vi "Log Result.vi"(8 "error in (no error)":errorcluster, 10 "tdms file":refnum<k34>, 11 "Scaled I32 Array Result in":refnum<class "Scaled I32 Array Result.lvclass">) -> (0 "error out":errorcluster, 2 "tdms file out":refnum<k34>, 3 "Scaled I32 Array Result out":refnum<class "Scaled I32 Array Result.lvclass">)   [LabVIEW 2015, in "Scaled I32 Array Result.lvclass"]
uses:
  Scaled I32 Array Result.lvclass
  Scaled I32 Array Result.lvclass/Scaled I32 Array Result.ctl
  Mag Lab Result.lvclass/Mag Lab Result.ctl
  Read Scale Array.vi
  Read Group Name.vi
  Read Channel names.vi
  Read I32 Array.vi
  <vilib>/Utility/tdmsutil.llb/TDMS Create Scaling Information (Linear).vi
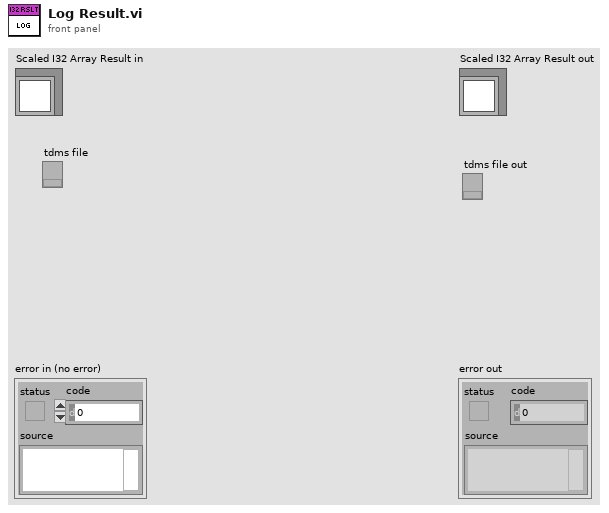
[diagram p1: front panel]
types:
  T1 = cluster{"Numeric":dbl, "Numeric":dbl, "input source":i32}
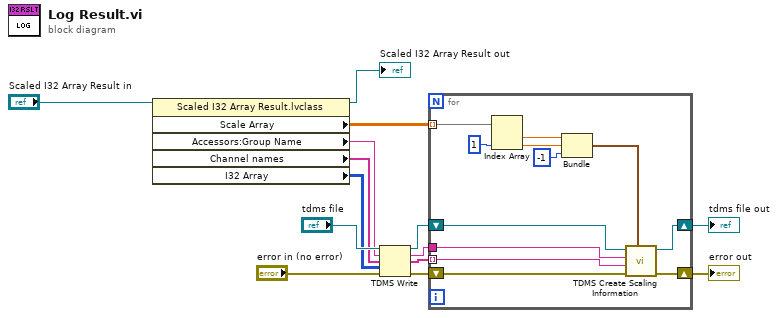
[diagram p0: block diagram]
diagram:
  n1 = property class="Scaled I32 Array Result.lvclass"(reference="Scaled I32 Array Result in") -> (reference out=→"Scaled I32 Array Result out":refnum<class "Scaled I32 Array Result.lvclass">, "Scale Array"=w5:dbl[][], "Accessors:Group Name"=w8:string, "Channel names"=w6:string[], "I32 Array"=w7:i32[][])  [unwired: 1 in, 1 out]
  n2 = TDMS Write(0:"tdms file", 5:w8, 7:w6, 9:w7, 11:"error in (no error)") -> (4:w4:refnum<k34>, 6:w9:string, 8:w10:string[], 15:w2:errorcluster)  [unwired: 1 in]
  n3 = for {
    tunnel: w10 -> [w26] mode=indexing
    tunnel: w9 -> [w25]
    tunnel: w5 -> [w24] mode=indexing
    shift-right: [w17] -> w3
    shift-left: w4 -> [w18]
    shift-right: [w15] -> w1
    shift-left: w2 -> [w16]
    n4 = Index Array(array=w24, index #2=1 ("index")) -> (element #1=w23:dbl, element #2=w22:dbl)  [unwired: 1 in]
    n5 = Bundle("Numeric"=w23, "Numeric"=w22, "input source"=-1) -> (w19:T1)  [unwired: 1 in]
    n6 = call-poly <vilib>:"TDMS Create Scaling Information.vi"("linear scale"=w19, "error in (no error)"=w16, "channel name"=w26, "group name"=w25, "tdms file"=w18) -> ("error out"=w15:errorcluster, "tdms file out"=w17:refnum<k34>)  [unwired: 2 in, 3 out]
  }
  "error out" <- w1
  "tdms file out" <- w3
